vi "Z900_navX_I2C_Read.vi"(8 "error in (no error)":errorcluster, 10 "Registry":u8[](array[numeric]), 11 "Interface TypeDefs":T1 {"I2CDevRef"."Device Address" format="%.0x"}) -> (0 "error out":errorcluster, 1 "Valid":bool, 2 "Registry":u8[](array[numeric]), 3 "Interface TypeDefs":T1 {"I2CDevRef"."Device Address" format="%.0x"})   [LabVIEW 2015, in "navX Library v2.lvlib"]
uses:
  navX Library v2.lvlib
  _TypeDefs/Z900_navX_InterfaceTypeDef.ctl
  <vilib>/Rock Robotics/WPI/SerialPort/WPI_SerialPortRef.ctl
  <vilib>/Rock Robotics/WPI/I2C/WPI_I2CDevRef.ctl
  <vilib>/Rock Robotics/SystemInterfaces/i2clib/i2c_bus.ctl
  <vilib>/Rock Robotics/WPI/SPI/WPI_SPIDevRef.ctl
  <vilib>/Rock Robotics/SystemInterfaces/spilib/spi_bus.ctl
  _TypeDefs/Z900_navX_DeviceRegisters.ctl
  _TypeDefs/Flags/Z900_navX_Flags_CapabilityTypeDef.ctl
  _Util/Z900_navX_Util_LittleEndian_to_BigEndian.vi
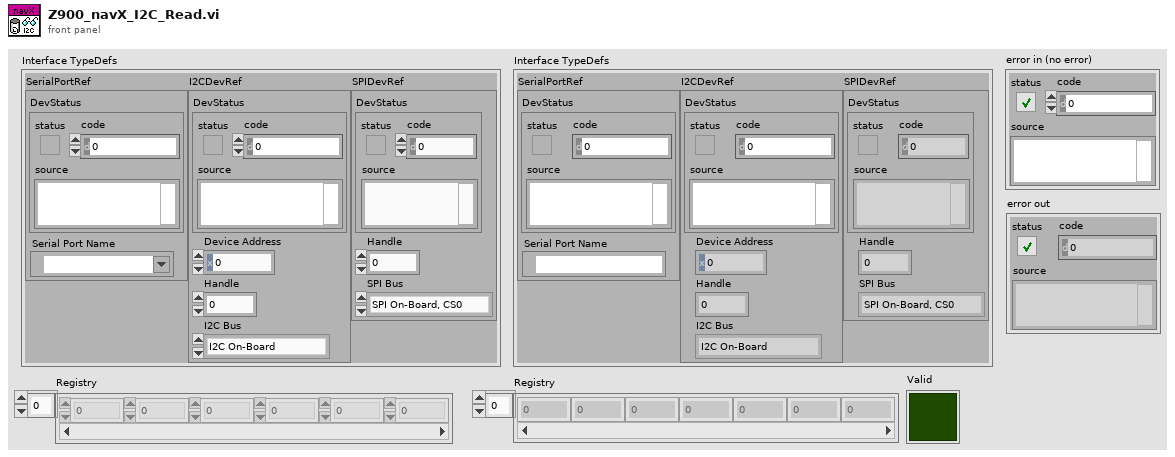
[diagram p1: front panel]
types:
  T1 = typedef "navX Library v2.lvlib/Z900_navX_InterfaceTypeDef.ctl" = cluster{"SerialPortRef":T2, "I2CDevRef":T3, "SPIDevRef":T5}
  T2 = typedef "WPI_SerialPortRef.ctl" = cluster{"DevStatus":errorcluster, "Serial Port Name":refnum<visa-resource-name>}
  T3 = typedef "WPI_I2CDevRef.ctl" = cluster{"DevStatus":errorcluster, "Device Address":u8, "Handle":i32, "I2C Bus":T4}
  T4 = typedef "i2c_bus.ctl" = enum16{"I2C On-Board", "I2C MXP", "Invalid"}
  T5 = typedef "WPI_SPIDevRef.ctl" = cluster{"DevStatus":errorcluster, "Handle":i32, "SPI Bus":T6}
  T6 = typedef "spi_bus.ctl" = enum16{"SPI On-Board, CS0", "SPI On-Board, CS1", "SPI On-Board, CS2", "SPI On-Board, CS3", "SPI MXP", "Invalid"}
  T7 = typedef "navX Library v2.lvlib/Z900_navX_Flags_CapabilityTypeDef.ctl" = u16
  T8 = typedef "navX Library v2.lvlib/Z900_navX_DeviceRegisters.ctl" = u8
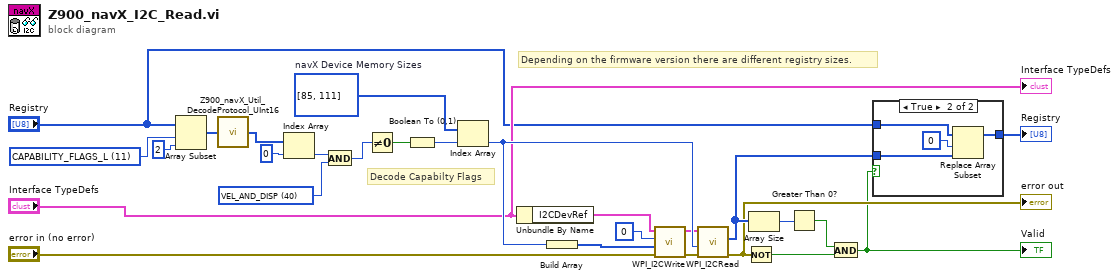
[diagram p0: block diagram]
diagram:
  w9 = T7 40 items=["OMNIMOUNT"=4, "OMNIMOUNT_CONFIG_MASK"=38, "VEL_AND_DISP"=40, "YAW_RESET"=80] ("Capability Flag")
  w11 = T8 11 items=["WHOAMI"=0, "HW_REV"=1, "FW_VER_MAJOR"=2, "FW_VER_MINOR"=3, "UPDATE_RATE_HZ"=4, "ACCEL_FSR_G"=5, "GYRO_FSR_DPS"=6, "OP_STATUS"=8, "CAL_STATUS"=9, "SELFTEST_STATUS"=10, "CAPABILITY_FLAGS_L"=11, "CAPABILITY_FLAGS_H"=12, "SENSOR_STATUS"=16, "TIMESTAMP"=18, "YAW"=22, "ROLL"=24, "PITCH"=26, "HEADING"=28, "FUSED_HEADING"=30, "ALTITUDE_I"=32, "ALTITUDE_D"=34, "LINERA_ACC_X"=36, "LINERA_ACC_Y"=38, "LINERA_ACC_Z"=40, "QUAT_W"=42, "QUAT_X"=44, "QUAT_Y"=46, "QUAT_Z"=48, "MPU_TEMP_C"=50, "GYRO_X"=52, "GYRO_Y"=54, "GYRO_Z"=56, "ACC_X"=58, "ACC_Y"=60, "ACC_Z"=62, "MAG_X"=64, "MAG_Y"=66, "MAG_Z"=68, "PRESSURE_I"=70, "PRESSURE_D"=72, "PRESSURE_TEMP"=74, "YAW_OFFSET"=76, "QUAT_OFFSET_W"=78, "QUAT_OFFSET_X"=80, "QUAT_OFFSET_Y"=82, "QUAT_OFFSET_Z"=84, "INTEGRATION_CONTROL"=86, "VELOCITY_X"=88, "VELOCITY_Y"=92, "VELOCITY_Z"=96, "DISPLACMENT_X"=100, "DISPLACMENT_Y"=104, "DISPLACEMENT_Z"=108] ("Device Register")
  w20 = i32[] [85, 111]  # navX Device Memory Sizes
  # "Decode Capabilty Flags"
  # "Depending on the firmware version there are different registry sizes."
  n1 = Array Subset(array="Registry", index=w11, length=2) -> (w15:u8[])
  n2 = call "Z900_navX_Util_DecodeProtocol_UInt16.vi"("Little Endian"=w15) -> ("UInt16"=w16:u16[])
  n3 = Index Array(array=w16, index=0) -> (element=w14:u16)
  n4 = And(x=w14, y=w9) -> (x .and. y?=w8:T7)
  n5 = Not Equal To 0?(x=w8) -> (x != 0?=w13:bool)
  n6 = Boolean To (0,1)(Boolean=w13) -> (0, 1=w12:i16)
  n7 = Index Array(array=w20, index=w12) -> (element=w25:i32)
  n8 = Unbundle By Name("Interface TypeDefs") -> ("I2CDevRef"=w26:T3)
  n9 = Build Array(w25) -> (w7:i32[])
  n10 = call <vilib>:"WPI_I2CWrite.vi"("error in (no error)"="error in (no error)", "I2CDataToSend"=w7, "I2CRegister"=u8 0 ("hex"), "I2CDevRef"=w26) -> ("error out"=w6:errorcluster, "I2CDevRef"=w5:T3)  [unwired: 6 in]
  n11 = call <vilib>:"WPI_I2CRead.vi"("error in (no error)"=w6, "I2CBytesToRead"=w25, "I2CDevRef"=w5) -> ("error out"=w22:errorcluster, "Data Out"=w27:u8[])  [unwired: 6 in, 1 out]
  "error out" <- w22
  n12 = Not(x=w22) -> (.not. x?=w1:bool)
  n13 = Array Size(array=w27) -> (size(s)=w3:i32)
  n14 = Greater Than 0?(x=w3) -> (x > 0?=w2:bool)
  n15 = And(x=w2, y=w1) -> (x .and. y?=w19:bool)
  "Valid" <- w19
  n16 = case shown="True" w19 {
    tunnel: "Registry" -> [w28 w32]
    tunnel: [w28 w31] -> w18
    tunnel: w27 -> [_ w30]
    frame False {
    }
    frame True {
      n17 = Replace Array Subset(array=w32, new element=w30, index=u8 0 ("hex")) -> (w31:u8[])
    }
  }
  "Registry" <- w18
  "Interface TypeDefs" <- "Interface TypeDefs"
